vi "autoTurn.vi"(10 "rightEncoderDesired":dbl, 11 "leftEncoderDesired":dbl) -> (3 "done?":bool)   [LabVIEW 2014]
uses:
  Robot Global Data.vi
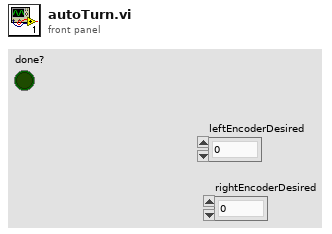
[diagram p1: front panel]
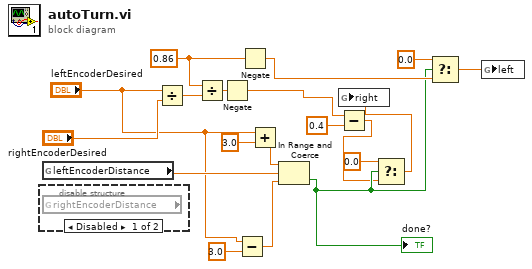
[diagram p0: block diagram]
diagram:
  w17 = 0.86
  n1 = disable-structure shown="Disabled" {
    frame Disabled {
      n2 = global read "Robot Global Data.vi" "rightEncoderDistance"() -> ()  [unwired: 1 out]
    }
    frame Enabled {
    }
  }
  n3 = global read "Robot Global Data.vi" "leftEncoderDistance"() -> (w15:dbl)
  n4 = Divide(x="leftEncoderDesired", y="rightEncoderDesired") -> (x/y=w18:dbl)
  n5 = Divide(x=w17, y=w18) -> (x/y=w16:dbl)
  n6 = Negate(x=w16) -> (-x=w4:dbl)
  n7 = Subtract(x="leftEncoderDesired", y=3.0) -> (x-y=w10:dbl)
  n8 = Negate(x=w17) -> (-x=w7:dbl)
  n9 = Add(x="leftEncoderDesired", y=3.0) -> (x+y=w13:dbl)
  n10 = In Range and Coerce(upper limit=w13, x=w15, lower limit=w10) -> (In Range?=w5:bool)  [unwired: 1 out]
  "done?" <- w5
  n11 = Subtract(x=w4, y=0.4) -> (x-y=w2:dbl)
  n12 = Select(t=0.0, s=w5, f=w2) -> (s? t:f=w1:dbl)
  n13 = global write "Robot Global Data.vi" "right"(w1) -> ()
  n14 = Select(t=0.0, s=w5, f=w7) -> (s? t:f=w6:dbl)
  n15 = global write "Robot Global Data.vi" "left"(w6) -> ()
